vi "Remove points in historam by threshold.vi"() -> ()   [LabVIEW 2023]
uses:
  <vilib>/Utility/file.llb/Read Delimited Spreadsheet (DBL).vi
  <vilib>/Utility/file.llb/Write Delimited Spreadsheet (DBL).vi
panel:
  in  "High pass?":bool
  in  "File name suffix":string(combo)="_reduced"
  in  "Threshold":dbl=1.0 format="%#_13g"
  out "Progress %":dbl=99.84375
  in  "book number":i32=821
  in  "file path (dialog if empty)":path=path "C:/Users/gyue/Desktop/GA01_202401"
  # "Remove data points smaller or larger than certain value"
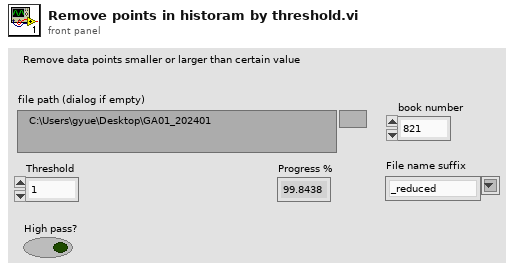
[diagram p1: front panel]
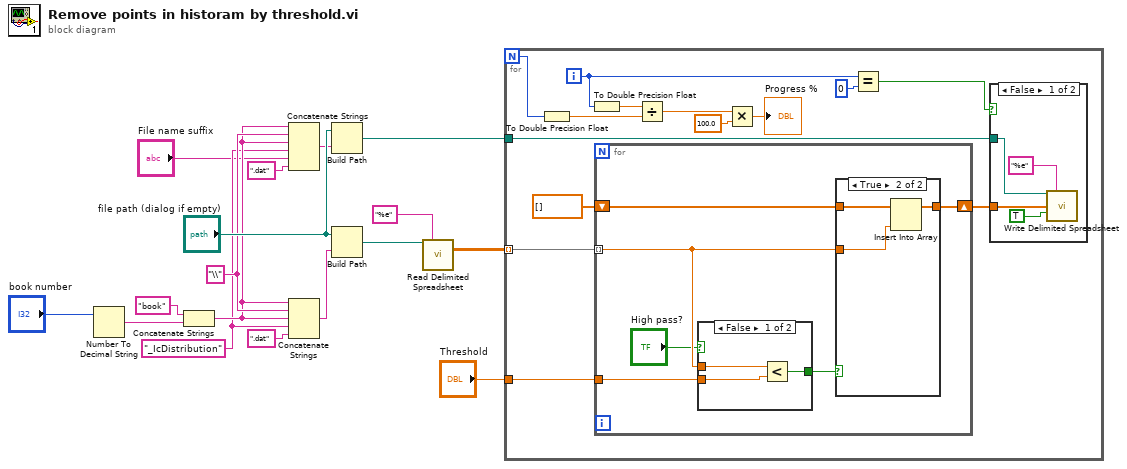
[diagram p0: block diagram]
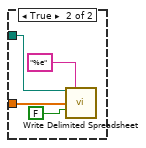
[diagram p2: hidden frame]
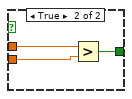
[diagram p3: hidden frame]
diagram:
  w6 = "_IcDistribution" ("string")
  w8 = "\\" ("string")
  n1 = Number To Decimal String(number="book number") -> (decimal integer string=w15:string)  [unwired: 1 in]
  n2 = Concatenate Strings("book" ("string"), w15) -> (w7:string)
  n3 = Concatenate Strings(w7, w8, w7, w6, "File name suffix", ".dat" ("string")) -> (w5:string)
  n4 = Concatenate Strings(w7, w8, w7, w6, ".dat" ("string")) -> (w16:string)
  n5 = Build Path(base path="file path (dialog if empty)", name or relative path=w5) -> (appended path=w4:path)
  n6 = Build Path(base path="file path (dialog if empty)", name or relative path=w16) -> (appended path=w17:path)
  n7 = call-poly <vilib>:"Read Delimited Spreadsheet.vi"("file path (dialog if empty)"=w17, "format (%.3f)"="%e") -> ("all rows"=w11:dbl[][])  [unwired: 8 in, 5 out]
  n8 = for {
    N -> [w31]
    tunnel: w11 -> [w27] mode=indexing
    tunnel: w4 -> [w20]
    tunnel: "Threshold" -> [w18]
    i -> [w25]
    n9 = To Double Precision Float(number=w31) -> (double precision float=w21:dbl)
    n10 = To Double Precision Float(number=w25) -> (double precision float=w22:dbl)
    n11 = for {
      tunnel: w27 -> [w43] mode=indexing
      shift-right: [w44] -> w19
      shift-left: dbl[] [] -> [w45]
      tunnel: w18 -> [w41]
      n12 = case shown="False" "High pass?" {
        tunnel: w43 -> [w48 w51]
        tunnel: [w46 w50] -> w42
        tunnel: w41 -> [w47 w49]
        frame False {
          n13 = Less?(x=w48, y=w47) -> (x < y?=w46:bool)
        }
        frame True {
          n14 = Greater?(x=w51, y=w49) -> (0:w50:bool)
        }
      }
      n15 = case shown="True" w42 {
        tunnel: w43 -> [_ w54]
        tunnel: w45 -> [w52 w55]
        tunnel: [w52 w53] -> w44
        frame False {
        }
        frame True {
          n16 = Insert Into Array(array=w55, new element=w54) -> (w53:dbl[])  [unwired: 1 in]
        }
      }
    }
    n17 = Divide(x=w22, y=w21) -> (x/y=w30:dbl)
    n18 = Multiply(x=w30, y=100.0) -> (x*y=→"Progress %":dbl)
    n19 = Equal?(x=w25, y=0) -> (x = y?=w23:bool)
    n20 = case shown="False" w23 {
      tunnel: w20 -> [w32 w39]
      tunnel: w19 -> [w33 w36]
      frame False {
        n21 = call-poly <vilib>:"Write Delimited Spreadsheet.vi"("file path (dialog if empty)"=w32, "format (%.3f)"="%e" ("format (%d)"), "1D data"=w33, "append to file? (new file:F)"=TRUE) -> ()  [unwired: 10 in, 2 out]
      }
      frame True {
        n22 = call-poly <vilib>:"Write Delimited Spreadsheet.vi"("file path (dialog if empty)"=w39, "format (%.3f)"="%e" ("format (%d)"), "1D data"=w36, "append to file? (new file:F)"=FALSE) -> ()  [unwired: 10 in, 2 out]
      }
    }
  }
